vi "XY Graph Compute Complex Plot Formula Event.vi"(8 "Error In":errorcluster, 11 "Mouse Click Event Data":T1) -> (0 "Error Out":errorcluster, 1 "Message":string, 2 "Formula":string, 3 "Plot Name":string, 5 "Graph Caption":string)   [LabVIEW 2021, in "XY Graph Add-Ons.lvlib"]
uses:
  XY Graph Add-Ons.lvlib
  XY Graph Mouse Click Event Data.ctl
  XY Graph Refnum.ctl
  <vilib>/Utility/miscctls.llb/LVPoint32TypeDef.ctl
  Get Plot at Mouse Click (XY Graph)/Get Plot at Mouse Click [AAC].vi
  XY Graph Add Single Plot with Name.vi
  Graphs.lvlib
  GUI/GUI.lvlib
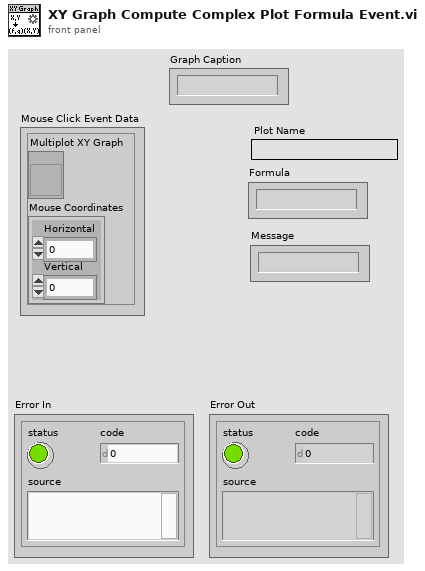
[diagram p1: front panel]
types:
  T1 = typedef "XY Graph Add-Ons.lvlib/XY Graph Mouse Click Event Data.ctl" = cluster{"Multiplot XY Graph":T2, "Mouse Coordinates":T3}
  T2 = typedef "XY Graph Add-Ons.lvlib/XY Graph Refnum.ctl" = refnum<vi>
  T3 = typedef "LVPoint32TypeDef.ctl" = cluster{"Horizontal":i32, "Vertical":i32}
  T4 = cluster{"f(X,Y) Array":dbl[], "g(X,Y) Array":dbl[]}
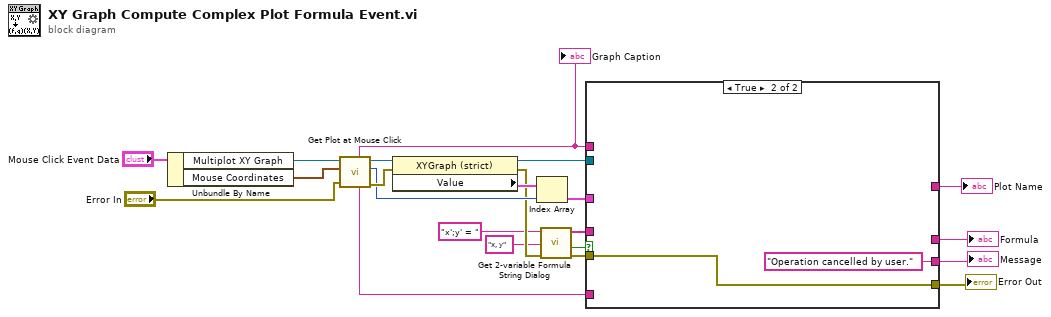
[diagram p0: block diagram]
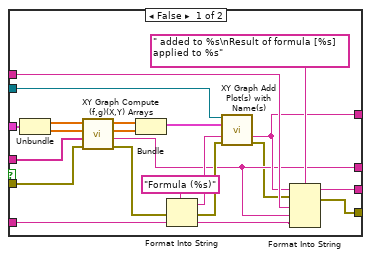
[diagram p2: hidden frame]
diagram:
  n1 = Unbundle By Name("Mouse Click Event Data") -> ("Multiplot XY Graph"=w21:T2, "Mouse Coordinates"=w20:T3)
  n2 = call-poly "Get Plot at Mouse Click.vi"("error in (no error)"="Error In", "Mouse Click Coordinates"=w20, "XYGraph Ref"=w21) -> ("error out"=w17:errorcluster, "Plot at Coordinates"=w15:i32, "XYGraph Ref"=w18:T2, "Plot Name"=w7:string, "Graph Name"=w6:string)  [unwired: 2 in, 2 out]
  "Graph Caption" <- w6
  n3 = property class="XYGraph (strict)"(reference=w18, error in=w17) -> (reference out=w10:T2, error out=w14:errorcluster, "Value"=w16:cluster{"X Array":dbl[], "Y Array":dbl[]}[])
  n4 = Index Array(array=w16, index=w15) -> (element=w13:cluster{"X Array":dbl[], "Y Array":dbl[]})
  n5 = call "Get 2-variable Formula String Dialog.vi"("error in (no error)"=w14, "Variables"="x, y", "Formula Names"="x';y' = ") -> ("error out"=w12:errorcluster, "Cancelled?"=w8:bool, "Formula"=w11:string[])  [unwired: 6 in]
  n6 = case shown="True" w8 {
    tunnel: w13 -> [w43 _]
    tunnel: w12 -> [w28 w45]
    tunnel: w11 -> [w26 _]
    tunnel: [w25 _] -> w3
    tunnel: w10 -> [w35 _]
    tunnel: [w23 w45] -> w9
    tunnel: w7 -> [w37 _]
    tunnel: w6 -> [w38 _]
    tunnel: [w36 "Operation cancelled by user."] -> w5
    tunnel: [w34 _] -> w4
    frame False {
      n7 = Unbundle(w43) -> ("X Array"=w33:dbl[], "Y Array"=w32:dbl[])
      n8 = call "XY Graph Compute (f,g)(X,Y) Arrays.vi"("Error In"=w28, "Formulas"=w26, "Y Array"=w32, "X Array"=w33) -> ("Error Out"=w27:errorcluster, "Formula String"=w25:string, "g(X,Y) Array"=w30:dbl[], "f(X,Y) Array"=w31:dbl[])  [unwired: 4 in]
      n9 = Bundle("f(X,Y) Array"=w31, "g(X,Y) Array"=w30) -> (w29:T4)  [unwired: 1 in]
      n10 = Format Into String(format string="Formula (%s)" ("initial string"), error in=w27, w37) -> (resulting string=w42:string, error out=w41:errorcluster)  [unwired: 1 in]
      n11 = call-poly "XY Graph Add Plot(s) with Name(s).vi"("XYGraph Ref in"=w35, "Plot"=w29, "Plot Name (\"Plot\")"=w42, "error in (no error)"=w41) -> ("Plot Name"=w34:string, "error out"=w24:errorcluster)  [unwired: 8 in, 2 out]
      n12 = Format Into String(format string=" added to %s\nResult of formula [%s] applied to %s", initial string=w34, error in=w24, w38, w25, w37) -> (resulting string=w36:string, error out=w23:errorcluster)
    }
    frame True {
    }
  }
  "Error Out" <- w9
  "Formula" <- w3
  "Message" <- w5
  "Plot Name" <- w4
